vi "Get VI Property.vi"(8 "error in (no error)":errorcluster, 10 "VI Property":T1, 11 "VI Refnum in":refnum<vi>) -> (0 "error out":errorcluster, 1 "Supported?":bool, 2 "Value":string, 3 "VI Refnum out":refnum<vi>)   [LabVIEW 2019, in "Project Properties.lvlib"]
doc: "Returns the <b>VI Property</b> as a string value. <b>Supported?</b> returns True if the property is accessable.\n\nCreated by: Ryan Pacini"
uses:
  Project Properties.lvlib
  VI Property.ctl
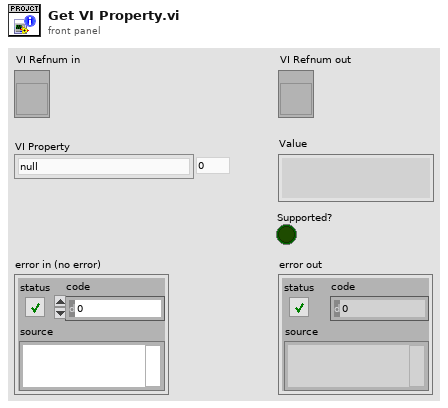
[diagram p1: front panel]
types:
  T1 = typedef "Project Properties.lvlib/VI Property.ctl" = enum8{"null", "Auto Logging:Log at Finish", "Auto Logging:Log File Path", "Auto Logging:Print at Finish", "Auto Preallocate Arrays and Strings", "Automatic Error Handling", "BD Master Wizard", "Block Diagram", "Block Diagram Window:Alignment Grid Size", "Block Diagram Window:Native Window", "Block Diagram Window:Open", "Block Diagram Window:Origin", "Block Diagram Window:State", "Block Diagram Window:Window Bounds", "Block Diagram Window:Window Interface", "Callers' Names", "Callers' Paths", "Compiled:Code Complexity", "Compiled:Last Compiled With", "Compiler:Generated Code Profiling Result", "Compiler:Generated Code Profiling Settings", "Connector Pane:Checksum Ignore Dynamic Dispatch v2", "Connector Pane:Checksum v3", "Connector Pane:DataType", "Connector Pane:Reference", "Connector Pane:Set", "Contains Compiled Code", "Context:Has Edits In Another Context", "Context:Has Edits In This Context", "Context:Is Reserved In Other Context", "Context:Is Reserved In This Context", "Control VI Type", "Did Recompile InThis Version", "Do Not Show Save Changes Dialog", "Edit Mode On Open", "Execution highlighting?", "Execution:Allow Debugging", "Execution:Close After Call", "Execution:Compiled With SSE", "Execution:Did Compiler Or User Approve Inlining", "Execution:Inline Enum", "Execution:Inline Is Allowed", "Execution:Inline SubVI", "Execution:Inline SubVI If Possible", "Execution:Is Reentrant", "Execution:Preferred Exec System", "Execution:Priority", "Execution:Reentrancy Type", "Execution:Retain Wire Values", "Execution:Run When Opened", "Execution:Show Front Panel On Call", "Execution:Show Front Panel On Load", "Execution:Shrink Large Buffer Threshold", "Execution:Shrink Large Buffers", "Execution:SSE Runtime Optimization", "Execution:State", "Execution:Suspend On Call", "Expand When Dropped As SubVI", "Front Panel", "Front Panel RefNum TD", "Front Panel Window:Alignment Grid Size", "Front Panel Window:Allow Runtime PopUp", "Front Panel Window:Behavior", "Front Panel Window:Closeable", "Front Panel Window:Custom Title", "Front Panel Window:Highlight Return Button", "Front Panel Window:Is Floating", "Front Panel Window:Is Frontmost", "Front Panel Window:Keep Window Proportions", "Front Panel Window:Minimizable", "Front Panel Window:Minimum Size", "Front Panel Window:Monitor", "Front Panel Window:Native Window", "Front Panel Window:Panel Bounds", "Front Panel Window:Resizable", "Front Panel Window:Run VI Transparently", "Front Panel Window:Show Menu Bar", "Front Panel Window:State", "Front Panel Window:Title", "Front Panel Window:Title Bar Visible", "Front Panel Window:Transparency", "Front Panel Window:Window Bounds", "Front Panel Window:Window Interface", "Has MathScript Nodes", "Help:Document Path", "Help:Document Tag", "Help:Document Web URL", "Help:Examples Exist", "Help:Use Web URL", "Hide Instance VI Caption On Drop", "History:Always Add Comments At Save", "History:Entire Text", "History:Prompt for Comments At Close", "History:Prompt for Comments At Save", "History:Record Application Comments", "History:Revision Number", "History:Use Defaults", "Inline Callees", "Is Clone VI", "Is Generic", "Is In Packed Library", "Is Instance", "Is Probe", "Is Running Interactively", "Is Skinned", "Is System VI", "Is VI Paused?", "Is XNode VI", "Item ID", "Ladder VI Needs Scripting", "Library", "Library:Private", "Library:Version", "Metrics:Advanced", "Metrics:Block Diagram Loaded", "Metrics:Code Size", "Metrics:Front Panel Loaded", "Metrics:Number of clones", "Metrics:Size of Block Diagram", "Metrics:Size of Front Panel", "Metrics:Total Data Size", "Modifications:Block Diagram Mods Bitset", "Modifications:Front Panel Mods Bitset", "Modifications:User Changes", "Modifications:VI Modifications Bitset", "Modifications:VI Signatures", "Modifications:VI User Code GUID", "No Clone If Instance VI", "Number of Non-Proxy Callers", "Overload Info", "Owning Application", "Printing:Block Diagram Scaling?", "Printing:Front Panel Scaling?", "Printing:Header Content:Date Printed?", "Printing:Header Content:Modify Date?", "Printing:Header Content:Page Number?", "Printing:Header Content:VI Icon?", "Printing:Header Content:VI Name?", "Printing:Header Content:VI Path?", "Printing:Margins", "Printing:Page Headers?", "Printing:Page Orientation", "Purgative", "Run-Time Menu Path", "Saved Version", "Statechart:Is Sub Panel Editable", "Statechart:Supress Parse", "Suppress Data Manager", "Suppress Instance VI Halo", "Suppress Transact Info", "Suppress Type Prop", "Tagged And Not Edited", "Terminal Bounds[]", "Tool Bar:Show Abort Button", "Tool Bar:Show Free Run Button", "Tool Bar:Show Run Button", "Tool Bar:Visible", "Tool Kit Attr", "VI Clone Name", "VI Compile Time", "VI Description", "VI Linker Errors", "VI Name", "VI Path", "VI Type"}
  T2 = typedef "LVPointTypeDef.ctl" = cluster{"Horizontal":i16, "Vertical":i16}
  T3 = enum32{"Invalid", "Standard", "Closed", "Hidden", "Minimized", "Maximized"}
  T4 = typedef "LVRectTypeDef.ctl" = cluster{"Left":i16, "Top":i16, "Right":i16, "Bottom":i16}
  T5 = typedef "LVLastCompiledWithTypeDef.ctl" = enum16{"Partial compiler optimizations", "Full compiler optimizations"}
  T6 = enum32{"not a control VI", "control", "typedef", "strict typedef"}
  T7 = enum32{"invalid execution system", "user interface", "standard", "instrument i/o", "data acquisition", "other 1", "other 2", "same as caller"}
  T8 = enum32{"invalid priority", "background priority", "normal priority", "above normal priority", "high priority", "time critical priority", "subroutine"}
  T9 = enum16{"Share clones between instances", "Preallocate clone for each instance"}
  T10 = enum32{"Bad", "Idle", "Run top level", "Running"}
  T11 = enum32{"Invalid", "Default", "Floating", "Floating/Auto-Hide", "Modal"}
  T12 = cluster{"Major":u16, "Minor":u16, "Fix":u16, "Build":u16}
  T13 = typedef "LVPrintingMarginsTypeDef.ctl" = cluster{"Top":sgl, "Left":sgl, "Bottom":sgl, "Right":sgl, "Measurement System":enum8{"Inches", "cm"}}
  T14 = enum32{"Portrait", "Landscape", "Rotated Portrait", "Rotated Landscape"}
  T15 = cluster{"Creator":string, "Toolkit":string, "Version":i32}
  T16 = enum32{"invalid VI type", "Standard VI", "Control VI", "Global VI", "Polymorphic VI", "Configuration VI", "SubSystem", "Facade VI", "Method VI", "Statechart Diagram VI"}
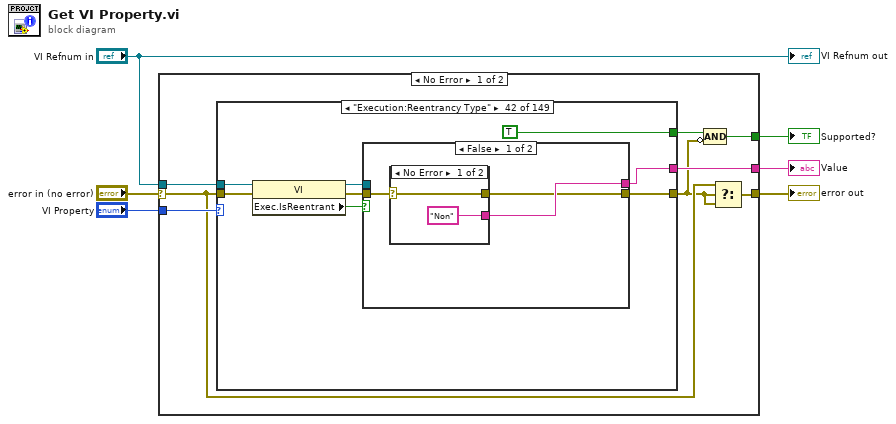
[diagram p0: block diagram]
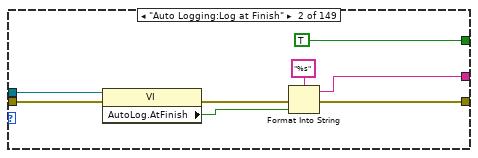
[diagram p3: hidden frame]
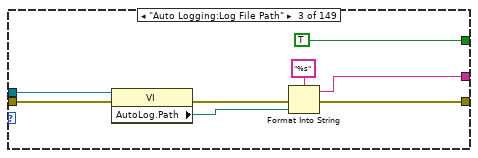
[diagram p4: hidden frame]
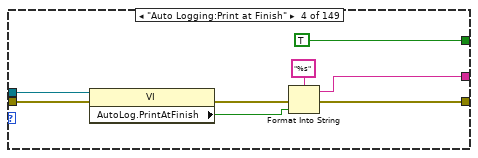
[diagram p5: hidden frame]
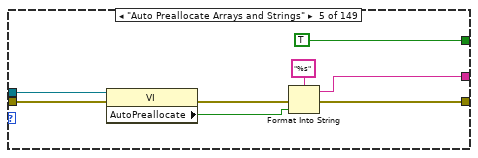
[diagram p6: hidden frame]
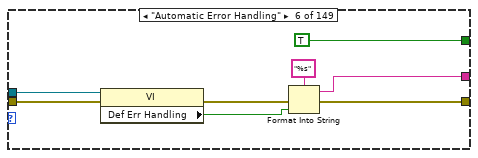
[diagram p7: hidden frame]
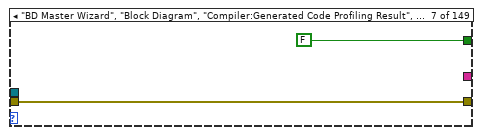
[diagram p8: hidden frame]
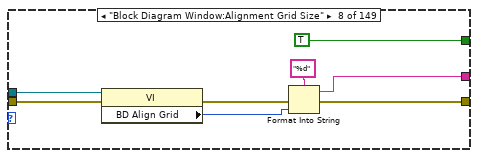
[diagram p9: hidden frame]
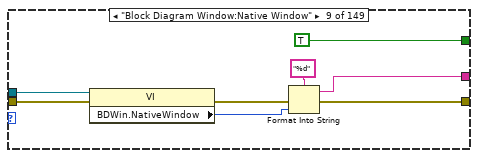
[diagram p10: hidden frame]
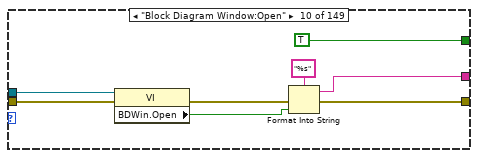
[diagram p11: hidden frame]
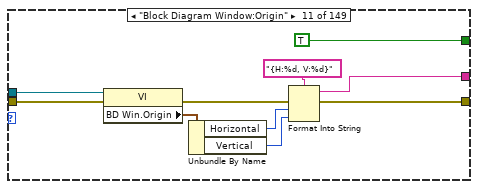
[diagram p12: hidden frame]
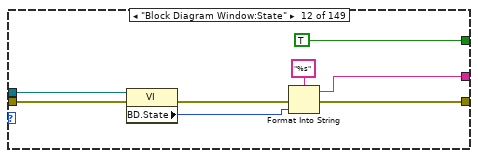
[diagram p13: hidden frame]
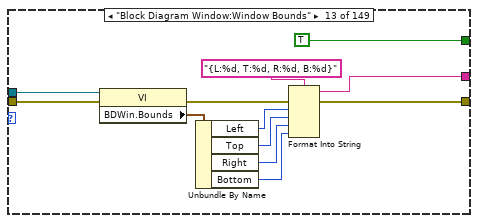
[diagram p14: hidden frame]
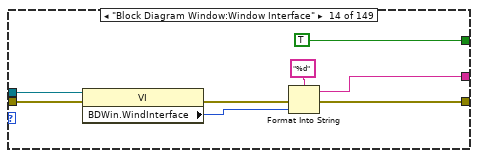
[diagram p15: hidden frame]
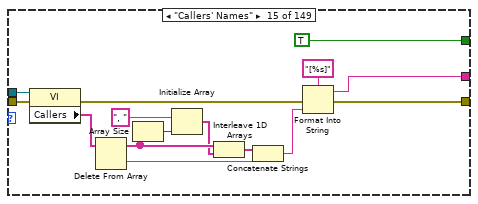
[diagram p16: hidden frame]
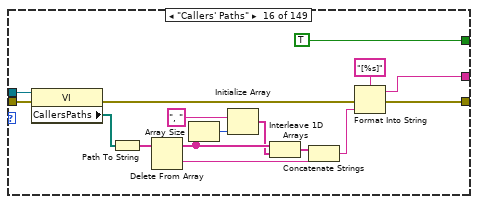
[diagram p17: hidden frame]
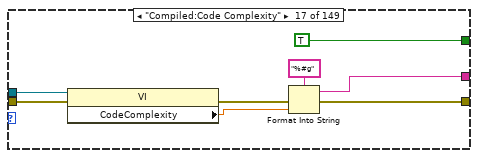
[diagram p18: hidden frame]
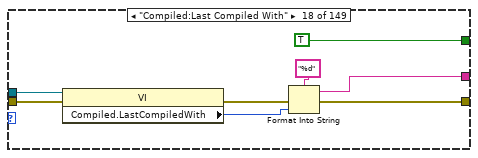
[diagram p19: hidden frame]
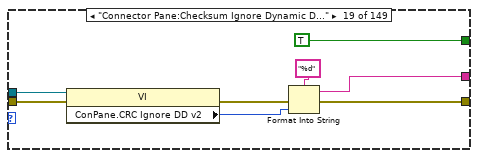
[diagram p20: hidden frame]
diagram:
  n1 = case shown="No Error" "error in (no error)" {
    selector: "error in (no error)" -> [w12 w1271]
    tunnel: "VI Property" -> [w14 _]
    tunnel: "VI Refnum in" -> [w13 _]
    tunnel: [w7 _] -> w3
    tunnel: [w11 w1271] -> w2
    tunnel: [w10 _] -> w1
    frame No Error {
      n2 = case shown="\"Execution:Reentrancy Type\"" w14 {
        tunnel: w12 -> [w15 w23 w31 w39 w47 w55 w56 w65 w73 w81 w91 w99 w111 w119 w134 w150 w158 w166 w174 w182 w190 w198 w206 w214 w222 w230 w238 w246 w254 w262 w270 w278 w286 w294 w302 w310 w318 w326 w334 w342 w350 w353 w382 w390 w398 w406 w414 w422 w430 w438 w446 w454 w462 w470 w478 w486 w494 w502 w510 w518 w526 w534 w544 w552 w560 w572 w580 w588 w596 w604 w612 w620 w628 w640 w648 w656 w664 w672 w680 w688 w696 w704 w712 w720 w728 w736 w744 w752 w760 w768 w776 w784 w792 w800 w808 w816 w824 w832 w840 w848 w856 w868 w876 w884 w892 w900 w908 w916 w924 w932 w940 w948 w956 w964 w972 w980 w988 w996 w1004 w1012 w1020 w1028 w1036 w1049 w1057 w1065 w1073 w1081 w1089 w1097 w1105 w1113 w1121 w1129 w1137 w1145 w1162 w1179 w1187 w1195 w1203 w1214 w1222 w1230 w1238 w1246 w1254 w1262 w1270]
        tunnel: w13 -> [_ w22 w30 w38 w46 w54 _ w64 w72 w80 w90 w98 w110 w118 w133 w149 w157 w165 w173 w181 w189 w197 w205 w213 w221 w229 w237 w245 w253 w261 w269 w277 w285 w293 w301 w309 w317 w325 w333 w341 w349 w358 w381 w389 w397 w405 w413 w421 w429 w437 w445 w453 w461 w469 w477 w485 w493 w501 w509 w517 w525 w533 w543 w551 w559 w571 w579 w587 w595 w603 w611 w619 w627 w639 w647 w655 w663 w671 w679 w687 w695 w703 w711 w719 w727 w735 w743 w751 w759 w767 w775 w783 w791 w799 w807 w815 w823 w831 w839 w847 w855 w867 w875 w883 w891 w899 w907 w915 w923 w931 w939 w947 w955 w963 w971 w979 w987 w995 w1003 w1011 w1019 w1027 w1035 w1048 w1056 w1064 w1072 w1080 w1088 w1096 w1104 w1112 w1120 w1128 w1136 w1144 w1161 w1178 w1186 w1194 w1202 w1213 w1221 w1229 w1237 w1245 w1253 w1261 w1269]
        tunnel: [w15 w19 w27 w35 w43 w51 w56 w61 w69 w77 w87 w95 w107 w115 w123 w138 w154 w162 w170 w178 w186 w194 w202 w210 w218 w226 w234 w242 w250 w258 w266 w274 w282 w290 w298 w306 w314 w322 w330 w338 w346 w356 w378 w386 w394 w402 w410 w418 w426 w434 w442 w450 w458 w466 w474 w482 w490 w498 w506 w514 w522 w530 w540 w548 w556 w568 w576 w584 w592 w600 w608 w616 w624 w636 w644 w652 w660 w668 w676 w684 w692 w700 w708 w716 w724 w732 w740 w748 w756 w764 w772 w780 w788 w796 w804 w812 w820 w828 w836 w844 w852 w864 w872 w880 w888 w896 w904 w912 w920 w928 w936 w944 w952 w960 w968 w976 w984 w992 w1000 w1008 w1016 w1024 w1032 w1045 w1053 w1061 w1069 w1077 w1085 w1093 w1101 w1109 w1117 w1125 w1133 w1141 w1150 w1175 w1183 w1191 w1199 w1210 w1218 w1226 w1234 w1242 w1250 w1258 w1266] -> w9
        tunnel: [_ TRUE TRUE TRUE TRUE TRUE FALSE TRUE TRUE TRUE TRUE TRUE TRUE TRUE TRUE TRUE TRUE TRUE TRUE TRUE TRUE TRUE TRUE TRUE TRUE TRUE TRUE TRUE TRUE TRUE TRUE TRUE TRUE TRUE TRUE TRUE TRUE TRUE TRUE TRUE TRUE TRUE TRUE TRUE TRUE TRUE TRUE TRUE TRUE TRUE TRUE TRUE TRUE TRUE TRUE TRUE TRUE TRUE TRUE TRUE TRUE TRUE TRUE TRUE TRUE TRUE TRUE TRUE TRUE TRUE TRUE TRUE TRUE TRUE TRUE TRUE TRUE TRUE TRUE TRUE TRUE TRUE TRUE TRUE TRUE TRUE TRUE TRUE TRUE TRUE TRUE TRUE TRUE TRUE TRUE TRUE TRUE TRUE TRUE TRUE TRUE TRUE TRUE TRUE TRUE TRUE TRUE TRUE TRUE TRUE TRUE TRUE TRUE TRUE TRUE TRUE TRUE TRUE TRUE TRUE TRUE TRUE TRUE TRUE TRUE TRUE TRUE TRUE TRUE TRUE TRUE TRUE TRUE TRUE TRUE TRUE TRUE TRUE TRUE TRUE TRUE TRUE TRUE TRUE TRUE TRUE TRUE TRUE TRUE] -> w8
        tunnel: [_ w16 w24 w32 w40 w48 _ w58 w66 w74 w85 w92 w105 w113 w121 w136 w152 w160 w168 w176 w184 w192 w200 w208 w216 w224 w232 w240 w248 w256 w264 w272 w280 w288 w296 w304 w312 w320 w328 w336 w344 w355 w376 w384 w392 w400 w408 w416 w424 w432 w440 w448 w456 w464 w472 w480 w488 w496 w504 w512 w520 w528 w538 w546 w554 w566 w574 w582 w590 w598 w606 w614 w622 w634 w642 w650 w658 w666 w674 w682 w690 w698 w706 w714 w722 w730 w738 w746 w754 w762 w770 w778 w786 w794 w802 w810 w818 w826 w834 w842 w850 w862 w870 w878 w886 w894 w902 w910 w918 w926 w934 w942 w950 w958 w966 w974 w982 w990 w998 w1006 w1014 w1022 w1030 w1043 w1051 w1059 w1067 w1075 w1083 w1091 w1099 w1107 w1115 w1123 w1131 w1139 w1148 w1173 w1181 w1189 w1197 w1208 w1216 w1224 w1232 w1240 w1248 w1256 w1264] -> w10
        frame "null" {
        }
        frame "Auto Logging:Log at Finish" {
          n3 = property class="VI"(reference=w22, error in=w23) -> (error out=w20:errorcluster, "AutoLog.AtFinish"=w18:bool)  [unwired: 1 out]
          n4 = Format Into String(format string="%s", error in=w20, w18) -> (resulting string=w16:string, error out=w19:errorcluster)  [unwired: 1 in]
        }
        frame "Auto Logging:Log File Path" {
          n5 = property class="VI"(reference=w30, error in=w31) -> (error out=w28:errorcluster, "AutoLog.Path"=w26:path)  [unwired: 1 out]
          n6 = Format Into String(format string="%s", error in=w28, w26) -> (resulting string=w24:string, error out=w27:errorcluster)  [unwired: 1 in]
        }
        frame "Auto Logging:Print at Finish" {
          n7 = property class="VI"(reference=w38, error in=w39) -> (error out=w36:errorcluster, "AutoLog.PrintAtFinish"=w34:bool)  [unwired: 1 out]
          n8 = Format Into String(format string="%s", error in=w36, w34) -> (resulting string=w32:string, error out=w35:errorcluster)  [unwired: 1 in]
        }
        frame "Auto Preallocate Arrays and Strings" {
          n9 = property class="VI"(reference=w46, error in=w47) -> (error out=w44:errorcluster, "AutoPreallocate"=w42:bool)  [unwired: 1 out]
          n10 = Format Into String(format string="%s", error in=w44, w42) -> (resulting string=w40:string, error out=w43:errorcluster)  [unwired: 1 in]
        }
        frame "Automatic Error Handling" {
          n11 = property class="VI"(reference=w54, error in=w55) -> (error out=w52:errorcluster, "Def Err Handling"=w50:bool)  [unwired: 1 out]
          n12 = Format Into String(format string="%s", error in=w52, w50) -> (resulting string=w48:string, error out=w51:errorcluster)  [unwired: 1 in]
        }
        frame "BD Master Wizard", "Block Diagram", "Compiler:Generated Code Profiling Result", "Compiler:Generated Code Profiling Settings", "Connector Pane:DataType".."Connector Pane:Set", "Front Panel", "Front Panel RefNum TD", "Inline Callees", "Library", "Library:Private", "Metrics:Advanced", "Modifications:VI Signatures", "Modifications:VI User Code GUID", "Overload Info", "Owning Application" {
        }
        frame "Block Diagram Window:Alignment Grid Size" {
          n13 = property class="VI"(reference=w64, error in=w65) -> (error out=w62:errorcluster, "BD Align Grid"=w60:i32)  [unwired: 1 out]
          n14 = Format Into String(format string="%d", error in=w62, w60) -> (resulting string=w58:string, error out=w61:errorcluster)  [unwired: 1 in]
        }
        frame "Block Diagram Window:Native Window" {
          n15 = property class="VI"(reference=w72, error in=w73) -> (error out=w70:errorcluster, "BDWin.NativeWindow"=w68:u64)  [unwired: 1 out]
          n16 = Format Into String(format string="%d", error in=w70, w68) -> (resulting string=w66:string, error out=w69:errorcluster)  [unwired: 1 in]
        }
        frame "Block Diagram Window:Open" {
          n17 = property class="VI"(reference=w80, error in=w81) -> (error out=w78:errorcluster, "BDWin.Open"=w76:bool)  [unwired: 1 out]
          n18 = Format Into String(format string="%s", error in=w78, w76) -> (resulting string=w74:string, error out=w77:errorcluster)  [unwired: 1 in]
        }
        frame "Block Diagram Window:Origin" {
          n19 = property class="VI"(reference=w90, error in=w91) -> (error out=w88:errorcluster, "BD Win.Origin"=w84:T2)  [unwired: 1 out]
          n20 = Unbundle By Name(w84) -> ("Horizontal"=w83:i16, "Vertical"=w82:i16)
          n21 = Format Into String(format string="{H:%d, V:%d}", error in=w88, w83, w82) -> (resulting string=w85:string, error out=w87:errorcluster)  [unwired: 1 in]
        }
        frame "Block Diagram Window:State" {
          n22 = property class="VI"(reference=w98, error in=w99) -> (error out=w96:errorcluster, "BD.State"=w94:T3)  [unwired: 1 out]
          n23 = Format Into String(format string="%s", error in=w96, w94) -> (resulting string=w92:string, error out=w95:errorcluster)  [unwired: 1 in]
        }
        frame "Block Diagram Window:Window Bounds" {
          n24 = property class="VI"(reference=w110, error in=w111) -> (error out=w108:errorcluster, "BDWin.Bounds"=w104:T4)  [unwired: 1 out]
          n25 = Unbundle By Name(w104) -> ("Left"=w103:i16, "Top"=w102:i16, "Right"=w101:i16, "Bottom"=w100:i16)
          n26 = Format Into String(format string="{L:%d, T:%d, R:%d, B:%d}", error in=w108, w103, w102, w101, w100) -> (resulting string=w105:string, error out=w107:errorcluster)  [unwired: 1 in]
        }
        frame "Block Diagram Window:Window Interface" {
          n27 = property class="VI"(reference=w118, error in=w119) -> (error out=w116:errorcluster, "BDWin.WindInterface"=w112:u64)  [unwired: 1 out]
          n28 = Format Into String(format string="%d", error in=w116, w112) -> (resulting string=w113:string, error out=w115:errorcluster)  [unwired: 1 in]
        }
        frame "Callers' Names" {
          n29 = property class="VI"(reference=w133, error in=w134) -> (error out=w124:errorcluster, "Callers"=w129:string[])  [unwired: 1 out]
          n30 = Delete From Array(array=w129) -> (deleted portion=w125:string, array with subset deleted=w128:string[])  [unwired: 2 in]
          n31 = Array Size(array=w128) -> (size(s)=w131:i32)
          n32 = Initialize Array(", ", w131) -> (w127:string[])
          n33 = Interleave 1D Arrays(w128, w127) -> (w126:string[])
          n34 = Concatenate Strings(w126, w125) -> (w122:string)
          n35 = Format Into String(format string="[%s]", error in=w124, w122) -> (resulting string=w121:string, error out=w123:errorcluster)  [unwired: 1 in]
        }
        frame "Callers' Paths" {
          n36 = property class="VI"(reference=w149, error in=w150) -> (error out=w140:errorcluster, "CallersPaths"=w145:path[])  [unwired: 1 out]
          n37 = Path To String(path=w145) -> (string=w139:string[])
          n38 = Delete From Array(array=w139) -> (deleted portion=w141:string, array with subset deleted=w144:string[])  [unwired: 2 in]
          n39 = Array Size(array=w144) -> (size(s)=w147:i32)
          n40 = Initialize Array(", ", w147) -> (w143:string[])
          n41 = Interleave 1D Arrays(w144, w143) -> (w142:string[])
          n42 = Concatenate Strings(w142, w141) -> (w137:string)
          n43 = Format Into String(format string="[%s]", error in=w140, w137) -> (resulting string=w136:string, error out=w138:errorcluster)  [unwired: 1 in]
        }
        frame "Compiled:Code Complexity" {
          n44 = property class="VI"(reference=w157, error in=w158) -> (error out=w155:errorcluster, "CodeComplexity"=w151:sgl)  [unwired: 1 out]
          n45 = Format Into String(format string="%#g", error in=w155, w151) -> (resulting string=w152:string, error out=w154:errorcluster)  [unwired: 1 in]
        }
        frame "Compiled:Last Compiled With" {
          n46 = property class="VI"(reference=w165, error in=w166) -> (error out=w163:errorcluster, "Compiled.LastCompiledWith"=w159:T5)  [unwired: 1 out]
          n47 = Format Into String(format string="%d", error in=w163, w159) -> (resulting string=w160:string, error out=w162:errorcluster)  [unwired: 1 in]
        }
        frame "Connector Pane:Checksum Ignore Dynamic Dispatch v2" {
          n48 = property class="VI"(reference=w173, error in=w174) -> (error out=w171:errorcluster, "ConPane.CRC Ignore DD v2"=w167:i32)  [unwired: 1 out]
          n49 = Format Into String(format string="%d", error in=w171, w167) -> (resulting string=w168:string, error out=w170:errorcluster)  [unwired: 1 in]
        }
        frame "Connector Pane:Checksum v3" {
          n50 = property class="VI"(reference=w181, error in=w182) -> (error out=w179:errorcluster, "ConPane.CRC v3"=w175:i32)  [unwired: 1 out]
          n51 = Format Into String(format string="%d", error in=w179, w175) -> (resulting string=w176:string, error out=w178:errorcluster)  [unwired: 1 in]
        }
        frame "Contains Compiled Code" {
          n52 = property class="VI"(reference=w189, error in=w190) -> (error out=w187:errorcluster, "ContainstCompiledCode"=w183:bool)  [unwired: 1 out]
          n53 = Format Into String(format string="%s", error in=w187, w183) -> (resulting string=w184:string, error out=w186:errorcluster)  [unwired: 1 in]
        }
        frame "Context:Has Edits In Another Context" {
          n54 = property class="VI"(reference=w197, error in=w198) -> (error out=w195:errorcluster, "HasEditsInAnotherContext"=w191:bool)  [unwired: 1 out]
          n55 = Format Into String(format string="%s", error in=w195, w191) -> (resulting string=w192:string, error out=w194:errorcluster)  [unwired: 1 in]
        }
        frame "Context:Has Edits In This Context" {
          n56 = property class="VI"(reference=w205, error in=w206) -> (error out=w203:errorcluster, "HasEditsInThisContext"=w199:bool)  [unwired: 1 out]
          n57 = Format Into String(format string="%s", error in=w203, w199) -> (resulting string=w200:string, error out=w202:errorcluster)  [unwired: 1 in]
        }
        frame "Context:Is Reserved In Other Context" {
          n58 = property class="VI"(reference=w213, error in=w214) -> (error out=w211:errorcluster, "IsReservedInOtherContext"=w207:bool)  [unwired: 1 out]
          n59 = Format Into String(format string="%s", error in=w211, w207) -> (resulting string=w208:string, error out=w210:errorcluster)  [unwired: 1 in]
        }
        frame "Context:Is Reserved In This Context" {
          n60 = property class="VI"(reference=w221, error in=w222) -> (error out=w219:errorcluster, "IsReservedInThisContext"=w215:bool)  [unwired: 1 out]
          n61 = Format Into String(format string="%s", error in=w219, w215) -> (resulting string=w216:string, error out=w218:errorcluster)  [unwired: 1 in]
        }
        frame "Control VI Type" {
          n62 = property class="VI"(reference=w229, error in=w230) -> (error out=w227:errorcluster, "CtrlVIType"=w223:T6)  [unwired: 1 out]
          n63 = Format Into String(format string="%s", error in=w227, w223) -> (resulting string=w224:string, error out=w226:errorcluster)  [unwired: 1 in]
        }
        frame "Did Recompile InThis Version" {
          n64 = property class="VI"(reference=w237, error in=w238) -> (error out=w235:errorcluster, "DidRecompileInThisVersion"=w231:bool)  [unwired: 1 out]
          n65 = Format Into String(format string="%s", error in=w235, w231) -> (resulting string=w232:string, error out=w234:errorcluster)  [unwired: 1 in]
        }
        frame "Do Not Show Save Changes Dialog" {
          n66 = property class="VI"(reference=w245, error in=w246) -> (error out=w243:errorcluster, "DoNotShowSaveChangesDialog"=w239:bool)  [unwired: 1 out]
          n67 = Format Into String(format string="%s", error in=w243, w239) -> (resulting string=w240:string, error out=w242:errorcluster)  [unwired: 1 in]
        }
        frame "Edit Mode On Open" {
          n68 = property class="VI"(reference=w253, error in=w254) -> (error out=w251:errorcluster, "Edit Mode"=w247:bool)  [unwired: 1 out]
          n69 = Format Into String(format string="%s", error in=w251, w247) -> (resulting string=w248:string, error out=w250:errorcluster)  [unwired: 1 in]
        }
        frame "Execution highlighting?" {
          n70 = property class="VI"(reference=w261, error in=w262) -> (error out=w259:errorcluster, "Highlight?"=w255:bool)  [unwired: 1 out]
          n71 = Format Into String(format string="%s", error in=w259, w255) -> (resulting string=w256:string, error out=w258:errorcluster)  [unwired: 1 in]
        }
        frame "Execution:Allow Debugging" {
          n72 = property class="VI"(reference=w269, error in=w270) -> (error out=w267:errorcluster, "Exec.AllowDebug"=w263:bool)  [unwired: 1 out]
          n73 = Format Into String(format string="%s", error in=w267, w263) -> (resulting string=w264:string, error out=w266:errorcluster)  [unwired: 1 in]
        }
        frame "Execution:Close After Call" {
          n74 = property class="VI"(reference=w277, error in=w278) -> (error out=w275:errorcluster, "Exec.CloseFPAfterCall"=w271:bool)  [unwired: 1 out]
          n75 = Format Into String(format string="%s", error in=w275, w271) -> (resulting string=w272:string, error out=w274:errorcluster)  [unwired: 1 in]
        }
        frame "Execution:Compiled With SSE" {
          n76 = property class="VI"(reference=w285, error in=w286) -> (error out=w283:errorcluster, "ExecCompiledWithSSE"=w279:bool)  [unwired: 1 out]
          n77 = Format Into String(format string="%s", error in=w283, w279) -> (resulting string=w280:string, error out=w282:errorcluster)  [unwired: 1 in]
        }
        frame "Execution:Did Compiler Or User Approve Inlining" {
          n78 = property class="VI"(reference=w293, error in=w294) -> (error out=w291:errorcluster, "Exec.DidCompilerOrUserApproveInlining"=w287:bool)  [unwired: 1 out]
          n79 = Format Into String(format string="%s", error in=w291, w287) -> (resulting string=w288:string, error out=w290:errorcluster)  [unwired: 1 in]
        }
        frame "Execution:Inline Enum" {
          n80 = property class="VI"(reference=w301, error in=w302) -> (error out=w299:errorcluster, "Exec.InlineSubVIEnum"=w295:u32)  [unwired: 1 out]
          n81 = Format Into String(format string="%d", error in=w299, w295) -> (resulting string=w296:string, error out=w298:errorcluster)  [unwired: 1 in]
        }
        frame "Execution:Inline Is Allowed" {
          n82 = property class="VI"(reference=w309, error in=w310) -> (error out=w307:errorcluster, "ExecIsInlineable"=w303:bool)  [unwired: 1 out]
          n83 = Format Into String(format string="%s", error in=w307, w303) -> (resulting string=w304:string, error out=w306:errorcluster)  [unwired: 1 in]
        }
        frame "Execution:Inline SubVI" {
          n84 = property class="VI"(reference=w317, error in=w318) -> (error out=w315:errorcluster, "ExecInlining"=w311:bool)  [unwired: 1 out]
          n85 = Format Into String(format string="%s", error in=w315, w311) -> (resulting string=w312:string, error out=w314:errorcluster)  [unwired: 1 in]
        }
        frame "Execution:Inline SubVI If Possible" {
          n86 = property class="VI"(reference=w325, error in=w326) -> (error out=w323:errorcluster, "ExecInlineIfPossible"=w319:bool)  [unwired: 1 out]
          n87 = Format Into String(format string="%s", error in=w323, w319) -> (resulting string=w320:string, error out=w322:errorcluster)  [unwired: 1 in]
        }
        frame "Execution:Is Reentrant" {
          n88 = property class="VI"(reference=w333, error in=w334) -> (error out=w331:errorcluster, "Exec.IsReentrant"=w327:bool)  [unwired: 1 out]
          n89 = Format Into String(format string="%s", error in=w331, w327) -> (resulting string=w328:string, error out=w330:errorcluster)  [unwired: 1 in]
        }
        frame "Execution:Preferred Exec System" {
          n90 = property class="VI"(reference=w341, error in=w342) -> (error out=w339:errorcluster, "Exec.PrefSys"=w335:T7)  [unwired: 1 out]
          n91 = Format Into String(format string="%s", error in=w339, w335) -> (resulting string=w336:string, error out=w338:errorcluster)  [unwired: 1 in]
        }
        frame "Execution:Priority" {
          n92 = property class="VI"(reference=w349, error in=w350) -> (error out=w347:errorcluster, "Exec.Priority"=w343:T8)  [unwired: 1 out]
          n93 = Format Into String(format string="%s", error in=w347, w343) -> (resulting string=w344:string, error out=w346:errorcluster)  [unwired: 1 in]
        }
        frame "Execution:Reentrancy Type" {
          n94 = property class="VI"(reference=w358, error in=w353) -> (reference out=w354:refnum<vi>, error out=w352:errorcluster, "Exec.IsReentrant"=w351:bool)
          n95 = case shown="False" w351 {
            tunnel: w352 -> [w359 w372]
            tunnel: w354 -> [_ w371]
            tunnel: [w360 w369] -> w356
            tunnel: [w361 w367] -> w355
            frame False {
              n96 = case shown="No Error" w359 {
                selector: w359 -> [w362 w364]
                tunnel: ["Non" _] -> w361
                tunnel: [w362 w364] -> w360
                frame No Error {
                }
                frame Error {
                }
              }
            }
            frame True {
              n97 = property class="VI"(reference=w371, error in=w372) -> (error out=w370:errorcluster, "Exec.ReentrancyType"=w366:T9)  [unwired: 1 out]
              n98 = case shown="\"Share clones between instances\"" w366 {
                tunnel: ["Share" ("format string") "Preallocate" ("format string")] -> w365
                frame "Share clones between instances" {
                }
                frame "Preallocate clone for each instance" {
                }
              }
              n99 = Format Into String(format string="%s", error in=w370, w365) -> (resulting string=w367:string, error out=w369:errorcluster)  [unwired: 1 in]
            }
          }
        }
        frame "Execution:Retain Wire Values" {
          n100 = property class="VI"(reference=w381, error in=w382) -> (error out=w379:errorcluster, "Exec.PostExecutionProbes"=w375:bool)  [unwired: 1 out]
          n101 = Format Into String(format string="%s", error in=w379, w375) -> (resulting string=w376:string, error out=w378:errorcluster)  [unwired: 1 in]
        }
        frame "Execution:Run When Opened" {
          n102 = property class="VI"(reference=w389, error in=w390) -> (error out=w387:errorcluster, "Exec.RunOnOpen"=w383:bool)  [unwired: 1 out]
          n103 = Format Into String(format string="%s", error in=w387, w383) -> (resulting string=w384:string, error out=w386:errorcluster)  [unwired: 1 in]
        }
        frame "Execution:Show Front Panel On Call" {
          n104 = property class="VI"(reference=w397, error in=w398) -> (error out=w395:errorcluster, "Exec.ShowFPOnCall"=w391:bool)  [unwired: 1 out]
          n105 = Format Into String(format string="%s", error in=w395, w391) -> (resulting string=w392:string, error out=w394:errorcluster)  [unwired: 1 in]
        }
        frame "Execution:Show Front Panel On Load" {
          n106 = property class="VI"(reference=w405, error in=w406) -> (error out=w403:errorcluster, "Exec.ShowFPOnLoad"=w399:bool)  [unwired: 1 out]
          n107 = Format Into String(format string="%s", error in=w403, w399) -> (resulting string=w400:string, error out=w402:errorcluster)  [unwired: 1 in]
        }
        frame "Execution:Shrink Large Buffer Threshold" {
          n108 = property class="VI"(reference=w413, error in=w414) -> (error out=w411:errorcluster, "Exec.ShrinkLargeBuffersThreshold"=w407:i32)  [unwired: 1 out]
          n109 = Format Into String(format string="%d", error in=w411, w407) -> (resulting string=w408:string, error out=w410:errorcluster)  [unwired: 1 in]
        }
        frame "Execution:Shrink Large Buffers" {
          n110 = property class="VI"(reference=w421, error in=w422) -> (error out=w419:errorcluster, "Exec.ShrinkLargeBuffers"=w415:bool)  [unwired: 1 out]
          n111 = Format Into String(format string="%s", error in=w419, w415) -> (resulting string=w416:string, error out=w418:errorcluster)  [unwired: 1 in]
        }
        frame "Execution:SSE Runtime Optimization" {
          n112 = property class="VI"(reference=w429, error in=w430) -> (error out=w427:errorcluster, "ExecSSERuntimeOptimization"=w423:bool)  [unwired: 1 out]
          n113 = Format Into String(format string="%s", error in=w427, w423) -> (resulting string=w424:string, error out=w426:errorcluster)  [unwired: 1 in]
        }
        frame "Execution:State" {
          n114 = property class="VI"(reference=w437, error in=w438) -> (error out=w435:errorcluster, "Exec.State"=w431:T10)  [unwired: 1 out]
          n115 = Format Into String(format string="%s", error in=w435, w431) -> (resulting string=w432:string, error out=w434:errorcluster)  [unwired: 1 in]
        }
        frame "Execution:Suspend On Call" {
          n116 = property class="VI"(reference=w445, error in=w446) -> (error out=w443:errorcluster, "Exec.SuspOnCall"=w439:bool)  [unwired: 1 out]
          n117 = Format Into String(format string="%s", error in=w443, w439) -> (resulting string=w440:string, error out=w442:errorcluster)  [unwired: 1 in]
        }
        frame "Expand When Dropped As SubVI" {
          n118 = property class="VI"(reference=w453, error in=w454) -> (error out=w451:errorcluster, "GrowByDefault"=w447:bool)  [unwired: 1 out]
          n119 = Format Into String(format string="%s", error in=w451, w447) -> (resulting string=w448:string, error out=w450:errorcluster)  [unwired: 1 in]
        }
        frame "Front Panel Window:Alignment Grid Size" {
          n120 = property class="VI"(reference=w461, error in=w462) -> (error out=w459:errorcluster, "FP Align Grid"=w455:i32)  [unwired: 1 out]
          n121 = Format Into String(format string="%d", error in=w459, w455) -> (resulting string=w456:string, error out=w458:errorcluster)  [unwired: 1 in]
        }
        frame "Front Panel Window:Allow Runtime PopUp" {
          n122 = property class="VI"(reference=w469, error in=w470) -> (error out=w467:errorcluster, "Front Panel.AllowRTPopup"=w463:bool)  [unwired: 1 out]
          n123 = Format Into String(format string="%d", error in=w467, w463) -> (resulting string=w464:string, error out=w466:errorcluster)  [unwired: 1 in]
        }
        frame "Front Panel Window:Behavior" {
          n124 = property class="VI"(reference=w477, error in=w478) -> (error out=w475:errorcluster, "FP.Behavior"=w471:T11)  [unwired: 1 out]
          n125 = Format Into String(format string="%d", error in=w475, w471) -> (resulting string=w472:string, error out=w474:errorcluster)  [unwired: 1 in]
        }
        frame "Front Panel Window:Closeable" {
          n126 = property class="VI"(reference=w485, error in=w486) -> (error out=w483:errorcluster, "Front Panel.Closeable"=w479:bool)  [unwired: 1 out]
          n127 = Format Into String(format string="%s", error in=w483, w479) -> (resulting string=w480:string, error out=w482:errorcluster)  [unwired: 1 in]
        }
        frame "Front Panel Window:Custom Title" {
          n128 = property class="VI"(reference=w493, error in=w494) -> (error out=w491:errorcluster, "Front Panel.CustomTitle"=w487:bool)  [unwired: 1 out]
          n129 = Format Into String(format string="%s", error in=w491, w487) -> (resulting string=w488:string, error out=w490:errorcluster)  [unwired: 1 in]
        }
        frame "Front Panel Window:Highlight Return Button" {
          n130 = property class="VI"(reference=w501, error in=w502) -> (error out=w499:errorcluster, "Front Panel.HiliteReturnBut"=w495:bool)  [unwired: 1 out]
          n131 = Format Into String(format string="%s", error in=w499, w495) -> (resulting string=w496:string, error out=w498:errorcluster)  [unwired: 1 in]
        }
        frame "Front Panel Window:Is Floating" {
          n132 = property class="VI"(reference=w509, error in=w510) -> (error out=w507:errorcluster, "FP.IsFloater"=w503:bool)  [unwired: 1 out]
          n133 = Format Into String(format string="%s", error in=w507, w503) -> (resulting string=w504:string, error out=w506:errorcluster)  [unwired: 1 in]
        }
        frame "Front Panel Window:Is Frontmost" {
          n134 = property class="VI"(reference=w517, error in=w518) -> (error out=w515:errorcluster, "Front Panel.IsFrontmost"=w511:bool)  [unwired: 1 out]
          n135 = Format Into String(format string="%s", error in=w515, w511) -> (resulting string=w512:string, error out=w514:errorcluster)  [unwired: 1 in]
        }
        frame "Front Panel Window:Keep Window Proportions" {
          n136 = property class="VI"(reference=w525, error in=w526) -> (error out=w523:errorcluster, "Front Panel.KeepWinProps"=w519:bool)  [unwired: 1 out]
          n137 = Format Into String(format string="%s", error in=w523, w519) -> (resulting string=w520:string, error out=w522:errorcluster)  [unwired: 1 in]
        }
        frame "Front Panel Window:Minimizable" {
          n138 = property class="VI"(reference=w533, error in=w534) -> (error out=w531:errorcluster, "Front Panel.Minimizeable"=w527:bool)  [unwired: 1 out]
          n139 = Format Into String(format string="%s", error in=w531, w527) -> (resulting string=w528:string, error out=w530:errorcluster)  [unwired: 1 in]
        }
        frame "Front Panel Window:Minimum Size" {
          n140 = property class="VI"(reference=w543, error in=w544) -> (error out=w541:errorcluster, "Minimum Panel Size"=w537:T2)  [unwired: 1 out]
          n141 = Unbundle By Name(w537) -> ("Horizontal"=w536:i16, "Vertical"=w535:i16)
          n142 = Format Into String(format string="{H:%d, V:%d}", error in=w541, w536, w535) -> (resulting string=w538:string, error out=w540:errorcluster)  [unwired: 1 in]
        }
        frame "Front Panel Window:Monitor" {
          n143 = property class="VI"(reference=w551, error in=w552) -> (error out=w549:errorcluster, "FP.Monitor"=w545:u16)  [unwired: 1 out]
          n144 = Format Into String(format string="%d", error in=w549, w545) -> (resulting string=w546:string, error out=w548:errorcluster)  [unwired: 1 in]
        }
        frame "Front Panel Window:Native Window" {
          n145 = property class="VI"(reference=w559, error in=w560) -> (error out=w557:errorcluster, "FP.NativeWindow"=w553:u64)  [unwired: 1 out]
          n146 = Format Into String(format string="%d", error in=w557, w553) -> (resulting string=w554:string, error out=w556:errorcluster)  [unwired: 1 in]
        }
        frame "Front Panel Window:Panel Bounds" {
          n147 = property class="VI"(reference=w571, error in=w572) -> (error out=w569:errorcluster, "Front Panel.PanelBounds"=w565:T4)  [unwired: 1 out]
          n148 = Unbundle By Name(w565) -> ("Left"=w564:i16, "Top"=w563:i16, "Right"=w562:i16, "Bottom"=w561:i16)
          n149 = Format Into String(format string="{L:%d, T:%d, R:%d, B:%d}", error in=w569, w564, w563, w562, w561) -> (resulting string=w566:string, error out=w568:errorcluster)  [unwired: 1 in]
        }
        frame "Front Panel Window:Resizable" {
          n150 = property class="VI"(reference=w579, error in=w580) -> (error out=w577:errorcluster, "Front Panel.Resizeable"=w573:bool)  [unwired: 1 out]
          n151 = Format Into String(format string="%s", error in=w577, w573) -> (resulting string=w574:string, error out=w576:errorcluster)  [unwired: 1 in]
        }
        frame "Front Panel Window:Run VI Transparently" {
          n152 = property class="VI"(reference=w587, error in=w588) -> (error out=w585:errorcluster, "FP:RunTransparently"=w581:bool)  [unwired: 1 out]
          n153 = Format Into String(format string="%s", error in=w585, w581) -> (resulting string=w582:string, error out=w584:errorcluster)  [unwired: 1 in]
        }
        frame "Front Panel Window:Show Menu Bar" {
          n154 = property class="VI"(reference=w595, error in=w596) -> (error out=w593:errorcluster, "Front Panel.ShowMenuBar"=w589:bool)  [unwired: 1 out]
          n155 = Format Into String(format string="%s", error in=w593, w589) -> (resulting string=w590:string, error out=w592:errorcluster)  [unwired: 1 in]
        }
        frame "Front Panel Window:State" {
          n156 = property class="VI"(reference=w603, error in=w604) -> (error out=w601:errorcluster, "FP.State"=w597:T3)  [unwired: 1 out]
          n157 = Format Into String(format string="%s", error in=w601, w597) -> (resulting string=w598:string, error out=w600:errorcluster)  [unwired: 1 in]
        }
        frame "Front Panel Window:Title" {
          n158 = property class="VI"(reference=w611, error in=w612) -> (error out=w609:errorcluster, "Front Panel.Title"=w605:string)  [unwired: 1 out]
          n159 = Format Into String(format string="%s", error in=w609, w605) -> (resulting string=w606:string, error out=w608:errorcluster)  [unwired: 1 in]
        }
        frame "Front Panel Window:Title Bar Visible" {
          n160 = property class="VI"(reference=w619, error in=w620) -> (error out=w617:errorcluster, "Front Panel.TitleBarVis"=w613:bool)  [unwired: 1 out]
          n161 = Format Into String(format string="%s", error in=w617, w613) -> (resulting string=w614:string, error out=w616:errorcluster)  [unwired: 1 in]
        }
        frame "Front Panel Window:Transparency" {
          n162 = property class="VI"(reference=w627, error in=w628) -> (error out=w625:errorcluster, "FP:Transparency"=w621:u8)  [unwired: 1 out]
          n163 = Format Into String(format string="%d", error in=w625, w621) -> (resulting string=w622:string, error out=w624:errorcluster)  [unwired: 1 in]
        }
        frame "Front Panel Window:Window Bounds" {
          n164 = property class="VI"(reference=w639, error in=w640) -> (error out=w637:errorcluster, "Front Panel.WinBounds"=w633:T4)  [unwired: 1 out]
          n165 = Unbundle By Name(w633) -> ("Left"=w632:i16, "Top"=w631:i16, "Right"=w630:i16, "Bottom"=w629:i16)
          n166 = Format Into String(format string="{L:%d, T:%d, R:%d, B:%d}", error in=w637, w632, w631, w630, w629) -> (resulting string=w634:string, error out=w636:errorcluster)  [unwired: 1 in]
        }
        frame "Front Panel Window:Window Interface" {
          n167 = property class="VI"(reference=w647, error in=w648) -> (error out=w645:errorcluster, "FP.WindInterface"=w641:u64)  [unwired: 1 out]
          n168 = Format Into String(format string="%d", error in=w645, w641) -> (resulting string=w642:string, error out=w644:errorcluster)  [unwired: 1 in]
        }
        frame "Has MathScript Nodes" {
          n169 = property class="VI"(reference=w655, error in=w656) -> (error out=w653:errorcluster, "HasMSN"=w649:bool)  [unwired: 1 out]
          n170 = Format Into String(format string="%s", error in=w653, w649) -> (resulting string=w650:string, error out=w652:errorcluster)  [unwired: 1 in]
        }
        frame "Help:Document Path" {
          n171 = property class="VI"(reference=w663, error in=w664) -> (error out=w661:errorcluster, "Help.Path"=w657:path)  [unwired: 1 out]
          n172 = Format Into String(format string="%s", error in=w661, w657) -> (resulting string=w658:string, error out=w660:errorcluster)  [unwired: 1 in]
        }
        frame "Help:Document Tag" {
          n173 = property class="VI"(reference=w671, error in=w672) -> (error out=w669:errorcluster, "Help.Tag"=w665:string)  [unwired: 1 out]
          n174 = Format Into String(format string="%s", error in=w669, w665) -> (resulting string=w666:string, error out=w668:errorcluster)  [unwired: 1 in]
        }
        frame "Help:Document Web URL" {
          n175 = property class="VI"(reference=w679, error in=w680) -> (error out=w677:errorcluster, "Help.URL"=w673:string)  [unwired: 1 out]
          n176 = Format Into String(format string="%s", error in=w677, w673) -> (resulting string=w674:string, error out=w676:errorcluster)  [unwired: 1 in]
        }
        frame "Help:Examples Exist" {
          n177 = property class="VI"(reference=w687, error in=w688) -> (error out=w685:errorcluster, "Help.Examples"=w681:bool)  [unwired: 1 out]
          n178 = Format Into String(format string="%s", error in=w685, w681) -> (resulting string=w682:string, error out=w684:errorcluster)  [unwired: 1 in]
        }
        frame "Help:Use Web URL" {
          n179 = property class="VI"(reference=w695, error in=w696) -> (error out=w693:errorcluster, "Help.UseOnline"=w689:bool)  [unwired: 1 out]
          n180 = Format Into String(format string="%s", error in=w693, w689) -> (resulting string=w690:string, error out=w692:errorcluster)  [unwired: 1 in]
        }
        frame "Hide Instance VI Caption On Drop" {
          n181 = property class="VI"(reference=w703, error in=w704) -> (error out=w701:errorcluster, "HideInstanceVICaptionOnDrop"=w697:bool)  [unwired: 1 out]
          n182 = Format Into String(format string="%s", error in=w701, w697) -> (resulting string=w698:string, error out=w700:errorcluster)  [unwired: 1 in]
        }
        frame "History:Always Add Comments At Save" {
          n183 = property class="VI"(reference=w711, error in=w712) -> (error out=w709:errorcluster, "Hist.AddAtSave"=w705:bool)  [unwired: 1 out]
          n184 = Format Into String(format string="%s", error in=w709, w705) -> (resulting string=w706:string, error out=w708:errorcluster)  [unwired: 1 in]
        }
        frame "History:Entire Text" {
          n185 = property class="VI"(reference=w719, error in=w720) -> (error out=w717:errorcluster, "Hist.Text"=w713:string)  [unwired: 1 out]
          n186 = Format Into String(format string="%s", error in=w717, w713) -> (resulting string=w714:string, error out=w716:errorcluster)  [unwired: 1 in]
        }
        frame "History:Prompt for Comments At Close" {
          n187 = property class="VI"(reference=w727, error in=w728) -> (error out=w725:errorcluster, "Hist.PromptAtClose"=w721:bool)  [unwired: 1 out]
          n188 = Format Into String(format string="%s", error in=w725, w721) -> (resulting string=w722:string, error out=w724:errorcluster)  [unwired: 1 in]
        }
        frame "History:Prompt for Comments At Save" {
          n189 = property class="VI"(reference=w735, error in=w736) -> (error out=w733:errorcluster, "Hist.PrompAtSave"=w729:bool)  [unwired: 1 out]
          n190 = Format Into String(format string="%s", error in=w733, w729) -> (resulting string=w730:string, error out=w732:errorcluster)  [unwired: 1 in]
        }
        frame "History:Record Application Comments" {
          n191 = property class="VI"(reference=w743, error in=w744) -> (error out=w741:errorcluster, "Hist.RecAppComments"=w737:bool)  [unwired: 1 out]
          n192 = Format Into String(format string="%s", error in=w741, w737) -> (resulting string=w738:string, error out=w740:errorcluster)  [unwired: 1 in]
        }
        frame "History:Revision Number" {
          n193 = property class="VI"(reference=w751, error in=w752) -> (error out=w749:errorcluster, "Hist.Revision"=w745:u32)  [unwired: 1 out]
          n194 = Format Into String(format string="%d", error in=w749, w745) -> (resulting string=w746:string, error out=w748:errorcluster)  [unwired: 1 in]
        }
        frame "History:Use Defaults" {
          n195 = property class="VI"(reference=w759, error in=w760) -> (error out=w757:errorcluster, "Hist.UseDflt"=w753:bool)  [unwired: 1 out]
          n196 = Format Into String(format string="%s", error in=w757, w753) -> (resulting string=w754:string, error out=w756:errorcluster)  [unwired: 1 in]
        }
        frame "Is Clone VI" {
          n197 = property class="VI"(reference=w767, error in=w768) -> (error out=w765:errorcluster, "IsCloneVI"=w761:bool)  [unwired: 1 out]
          n198 = Format Into String(format string="%s", error in=w765, w761) -> (resulting string=w762:string, error out=w764:errorcluster)  [unwired: 1 in]
        }
        frame "Is Generic" {
          n199 = property class="VI"(reference=w775, error in=w776) -> (error out=w773:errorcluster, "IsGeneric"=w769:bool)  [unwired: 1 out]
          n200 = Format Into String(format string="%s", error in=w773, w769) -> (resulting string=w770:string, error out=w772:errorcluster)  [unwired: 1 in]
        }
        frame "Is In Packed Library" {
          n201 = property class="VI"(reference=w783, error in=w784) -> (error out=w781:errorcluster, "IsInPackedLibrary"=w777:bool)  [unwired: 1 out]
          n202 = Format Into String(format string="%s", error in=w781, w777) -> (resulting string=w778:string, error out=w780:errorcluster)  [unwired: 1 in]
        }
        frame "Is Instance" {
          n203 = property class="VI"(reference=w791, error in=w792) -> (error out=w789:errorcluster, "Is Instance ?"=w785:bool)  [unwired: 1 out]
          n204 = Format Into String(format string="%s", error in=w789, w785) -> (resulting string=w786:string, error out=w788:errorcluster)  [unwired: 1 in]
        }
        frame "Is Probe" {
          n205 = property class="VI"(reference=w799, error in=w800) -> (error out=w797:errorcluster, "IsSmartProbe"=w793:bool)  [unwired: 1 out]
          n206 = Format Into String(format string="%s", error in=w797, w793) -> (resulting string=w794:string, error out=w796:errorcluster)  [unwired: 1 in]
        }
        frame "Is Running Interactively" {
          n207 = property class="VI"(reference=w807, error in=w808) -> (error out=w805:errorcluster, "HasRemoteObservers"=w801:bool)  [unwired: 1 out]
          n208 = Format Into String(format string="%s", error in=w805, w801) -> (resulting string=w802:string, error out=w804:errorcluster)  [unwired: 1 in]
        }
        frame "Is Skinned" {
          n209 = property class="VI"(reference=w815, error in=w816) -> (error out=w813:errorcluster, "IsSkinned"=w809:bool)  [unwired: 1 out]
          n210 = Format Into String(format string="%s", error in=w813, w809) -> (resulting string=w810:string, error out=w812:errorcluster)  [unwired: 1 in]
        }
        frame "Is System VI" {
          n211 = property class="VI"(reference=w823, error in=w824) -> (error out=w821:errorcluster, "IsSystemVI"=w817:bool)  [unwired: 1 out]
          n212 = Format Into String(format string="%s", error in=w821, w817) -> (resulting string=w818:string, error out=w820:errorcluster)  [unwired: 1 in]
        }
        frame "Is VI Paused?" {
          n213 = property class="VI"(reference=w831, error in=w832) -> (error out=w829:errorcluster, "Is VI Paused?"=w825:bool)  [unwired: 1 out]
          n214 = Format Into String(format string="%s", error in=w829, w825) -> (resulting string=w826:string, error out=w828:errorcluster)  [unwired: 1 in]
        }
        frame "Is XNode VI" {
          n215 = property class="VI"(reference=w839, error in=w840) -> (error out=w837:errorcluster, "X VI"=w833:bool)  [unwired: 1 out]
          n216 = Format Into String(format string="%s", error in=w837, w833) -> (resulting string=w834:string, error out=w836:errorcluster)  [unwired: 1 in]
        }
        frame "Item ID" {
          n217 = property class="VI"(reference=w847, error in=w848) -> (error out=w845:errorcluster, "ItemID"=w841:string)  [unwired: 1 out]
          n218 = Format Into String(format string="%s", error in=w845, w841) -> (resulting string=w842:string, error out=w844:errorcluster)  [unwired: 1 in]
        }
        frame "Ladder VI Needs Scripting" {
          n219 = property class="VI"(reference=w855, error in=w856) -> (error out=w853:errorcluster, "LadderVINeedsScripting"=w849:bool)  [unwired: 1 out]
          n220 = Format Into String(format string="%s", error in=w853, w849) -> (resulting string=w850:string, error out=w852:errorcluster)  [unwired: 1 in]
        }
        frame "Library:Version" {
          n221 = property class="VI"(reference=w867, error in=w868) -> (error out=w865:errorcluster, "Library.Version"=w861:T12)  [unwired: 1 out]
          n222 = Unbundle By Name(w861) -> ("Major"=w860:u16, "Minor"=w859:u16, "Fix"=w858:u16, "Build"=w857:u16)
          n223 = Format Into String(format string="%d.%d.%d.%d", error in=w865, w860, w859, w858, w857) -> (resulting string=w862:string, error out=w864:errorcluster)  [unwired: 1 in]
        }
        frame "Metrics:Block Diagram Loaded" {
          n224 = property class="VI"(reference=w875, error in=w876) -> (error out=w873:errorcluster, "DiagramLoaded"=w869:bool)  [unwired: 1 out]
          n225 = Format Into String(format string="%s", error in=w873, w869) -> (resulting string=w870:string, error out=w872:errorcluster)  [unwired: 1 in]
        }
        frame "Metrics:Code Size" {
          n226 = property class="VI"(reference=w883, error in=w884) -> (error out=w881:errorcluster, "Metric.CodeSize"=w877:u32)  [unwired: 1 out]
          n227 = Format Into String(format string="%d", error in=w881, w877) -> (resulting string=w878:string, error out=w880:errorcluster)  [unwired: 1 in]
        }
        frame "Metrics:Front Panel Loaded" {
          n228 = property class="VI"(reference=w891, error in=w892) -> (error out=w889:errorcluster, "PanelLoaded"=w885:bool)  [unwired: 1 out]
          n229 = Format Into String(format string="%s", error in=w889, w885) -> (resulting string=w886:string, error out=w888:errorcluster)  [unwired: 1 in]
        }
        frame "Metrics:Number of clones" {
          n230 = property class="VI"(reference=w899, error in=w900) -> (error out=w897:errorcluster, "Metric.NumberOfClones"=w893:u32)  [unwired: 1 out]
          n231 = Format Into String(format string="%d", error in=w897, w893) -> (resulting string=w894:string, error out=w896:errorcluster)  [unwired: 1 in]
        }
        frame "Metrics:Size of Block Diagram" {
          n232 = property class="VI"(reference=w907, error in=w908) -> (error out=w905:errorcluster, "Metric.BDSize"=w901:u32)  [unwired: 1 out]
          n233 = Format Into String(format string="%d", error in=w905, w901) -> (resulting string=w902:string, error out=w904:errorcluster)  [unwired: 1 in]
        }
        frame "Metrics:Size of Front Panel" {
          n234 = property class="VI"(reference=w915, error in=w916) -> (error out=w913:errorcluster, "Metric.FPSize"=w909:u32)  [unwired: 1 out]
          n235 = Format Into String(format string="%d", error in=w913, w909) -> (resulting string=w910:string, error out=w912:errorcluster)  [unwired: 1 in]
        }
        frame "Metrics:Total Data Size" {
          n236 = property class="VI"(reference=w923, error in=w924) -> (error out=w921:errorcluster, "Metric.DataSize"=w917:u32)  [unwired: 1 out]
          n237 = Format Into String(format string="%d", error in=w921, w917) -> (resulting string=w918:string, error out=w920:errorcluster)  [unwired: 1 in]
        }
        frame "Modifications:Block Diagram Mods Bitset" {
          n238 = property class="VI"(reference=w931, error in=w932) -> (error out=w929:errorcluster, "Mods.Block Diagram"=w925:u32)  [unwired: 1 out]
          n239 = Format Into String(format string="%d", error in=w929, w925) -> (resulting string=w926:string, error out=w928:errorcluster)  [unwired: 1 in]
        }
        frame "Modifications:Front Panel Mods Bitset" {
          n240 = property class="VI"(reference=w939, error in=w940) -> (error out=w937:errorcluster, "Mods.Front Panel"=w933:u32)  [unwired: 1 out]
          n241 = Format Into String(format string="%d", error in=w937, w933) -> (resulting string=w934:string, error out=w936:errorcluster)  [unwired: 1 in]
        }
        frame "Modifications:User Changes" {
          n242 = property class="VI"(reference=w947, error in=w948) -> (error out=w945:errorcluster, "Mods.User Changes"=w941:bool)  [unwired: 1 out]
          n243 = Format Into String(format string="%s", error in=w945, w941) -> (resulting string=w942:string, error out=w944:errorcluster)  [unwired: 1 in]
        }
        frame "Modifications:VI Modifications Bitset" {
          n244 = property class="VI"(reference=w955, error in=w956) -> (error out=w953:errorcluster, "Mods.VI"=w949:u64)  [unwired: 1 out]
          n245 = Format Into String(format string="%d", error in=w953, w949) -> (resulting string=w950:string, error out=w952:errorcluster)  [unwired: 1 in]
        }
        frame "No Clone If Instance VI" {
          n246 = property class="VI"(reference=w963, error in=w964) -> (error out=w961:errorcluster, "NoCloneIfInstanceVI"=w957:bool)  [unwired: 1 out]
          n247 = Format Into String(format string="%s", error in=w961, w957) -> (resulting string=w958:string, error out=w960:errorcluster)  [unwired: 1 in]
        }
        frame "Number of Non-Proxy Callers" {
          n248 = property class="VI"(reference=w971, error in=w972) -> (error out=w969:errorcluster, "NonProxyCallers"=w965:i32)  [unwired: 1 out]
          n249 = Format Into String(format string="%d", error in=w969, w965) -> (resulting string=w966:string, error out=w968:errorcluster)  [unwired: 1 in]
        }
        frame "Printing:Block Diagram Scaling?" {
          n250 = property class="VI"(reference=w979, error in=w980) -> (error out=w977:errorcluster, "Printing.BDScaling"=w973:bool)  [unwired: 1 out]
          n251 = Format Into String(format string="%s", error in=w977, w973) -> (resulting string=w974:string, error out=w976:errorcluster)  [unwired: 1 in]
        }
        frame "Printing:Front Panel Scaling?" {
          n252 = property class="VI"(reference=w987, error in=w988) -> (error out=w985:errorcluster, "Printing.FPScaling"=w981:bool)  [unwired: 1 out]
          n253 = Format Into String(format string="%s", error in=w985, w981) -> (resulting string=w982:string, error out=w984:errorcluster)  [unwired: 1 in]
        }
        frame "Printing:Header Content:Date Printed?" {
          n254 = property class="VI"(reference=w995, error in=w996) -> (error out=w993:errorcluster, "Print.Header Content.Date Printed"=w989:bool)  [unwired: 1 out]
          n255 = Format Into String(format string="%s", error in=w993, w989) -> (resulting string=w990:string, error out=w992:errorcluster)  [unwired: 1 in]
        }
        frame "Printing:Header Content:Modify Date?" {
          n256 = property class="VI"(reference=w1003, error in=w1004) -> (error out=w1001:errorcluster, "Print.Header Content.Modify Date"=w997:bool)  [unwired: 1 out]
          n257 = Format Into String(format string="%s", error in=w1001, w997) -> (resulting string=w998:string, error out=w1000:errorcluster)  [unwired: 1 in]
        }
        frame "Printing:Header Content:Page Number?" {
          n258 = property class="VI"(reference=w1011, error in=w1012) -> (error out=w1009:errorcluster, "Print.Header Content.Page Number"=w1005:bool)  [unwired: 1 out]
          n259 = Format Into String(format string="%s", error in=w1009, w1005) -> (resulting string=w1006:string, error out=w1008:errorcluster)  [unwired: 1 in]
        }
        frame "Printing:Header Content:VI Icon?" {
          n260 = property class="VI"(reference=w1019, error in=w1020) -> (error out=w1017:errorcluster, "Print.Header Content.VIIcon"=w1013:bool)  [unwired: 1 out]
          n261 = Format Into String(format string="%s", error in=w1017, w1013) -> (resulting string=w1014:string, error out=w1016:errorcluster)  [unwired: 1 in]
        }
        frame "Printing:Header Content:VI Name?" {
          n262 = property class="VI"(reference=w1027, error in=w1028) -> (error out=w1025:errorcluster, "Printing.HeaderContent.VIName"=w1021:bool)  [unwired: 1 out]
          n263 = Format Into String(format string="%s", error in=w1025, w1021) -> (resulting string=w1022:string, error out=w1024:errorcluster)  [unwired: 1 in]
        }
        frame "Printing:Header Content:VI Path?" {
          n264 = property class="VI"(reference=w1035, error in=w1036) -> (error out=w1033:errorcluster, "Printing.Header Content.VIPath"=w1029:bool)  [unwired: 1 out]
          n265 = Format Into String(format string="%s", error in=w1033, w1029) -> (resulting string=w1030:string, error out=w1032:errorcluster)  [unwired: 1 in]
        }
        frame "Printing:Margins" {
          n266 = property class="VI"(reference=w1048, error in=w1049) -> (error out=w1046:errorcluster, "Printing.Margin"=w1042:T13)  [unwired: 1 out]
          n267 = Unbundle By Name(w1042) -> ("Top"=w1040:sgl, "Left"=w1041:sgl, "Bottom"=w1038:sgl, "Right"=w1039:sgl, "Measurement System"=w1037:enum8{"Inches", "cm"})
          n268 = Format Into String(format string="{L:%#g, T:%#g, R:%#g, B:%#g, U:%s}", error in=w1046, w1041, w1040, w1039, w1038, w1037) -> (resulting string=w1043:string, error out=w1045:errorcluster)  [unwired: 1 in]
        }
        frame "Printing:Page Headers?" {
          n269 = property class="VI"(reference=w1056, error in=w1057) -> (error out=w1054:errorcluster, "Printing.Headers"=w1050:bool)  [unwired: 1 out]
          n270 = Format Into String(format string="%s", error in=w1054, w1050) -> (resulting string=w1051:string, error out=w1053:errorcluster)  [unwired: 1 in]
        }
        frame "Printing:Page Orientation" {
          n271 = property class="VI"(reference=w1064, error in=w1065) -> (error out=w1062:errorcluster, "Printing.Orientation"=w1058:T14)  [unwired: 1 out]
          n272 = Format Into String(format string="%s", error in=w1062, w1058) -> (resulting string=w1059:string, error out=w1061:errorcluster)  [unwired: 1 in]
        }
        frame "Purgative" {
          n273 = property class="VI"(reference=w1072, error in=w1073) -> (error out=w1070:errorcluster, "Purgative"=w1066:bool)  [unwired: 1 out]
          n274 = Format Into String(format string="%s", error in=w1070, w1066) -> (resulting string=w1067:string, error out=w1069:errorcluster)  [unwired: 1 in]
        }
        frame "Run-Time Menu Path" {
          n275 = property class="VI"(reference=w1080, error in=w1081) -> (error out=w1078:errorcluster, "RT Menu Path"=w1074:path)  [unwired: 1 out]
          n276 = Format Into String(format string="%s", error in=w1078, w1074) -> (resulting string=w1075:string, error out=w1077:errorcluster)  [unwired: 1 in]
        }
        frame "Saved Version" {
          n277 = property class="VI"(reference=w1088, error in=w1089) -> (error out=w1086:errorcluster, "SavedVersion"=w1082:u32)  [unwired: 1 out]
          n278 = Format Into String(format string="%d", error in=w1086, w1082) -> (resulting string=w1083:string, error out=w1085:errorcluster)  [unwired: 1 in]
        }
        frame "Statechart:Is Sub Panel Editable" {
          n279 = property class="VI"(reference=w1096, error in=w1097) -> (error out=w1094:errorcluster, "IsSCEditable"=w1090:bool)  [unwired: 1 out]
          n280 = Format Into String(format string="%s", error in=w1094, w1090) -> (resulting string=w1091:string, error out=w1093:errorcluster)  [unwired: 1 in]
        }
        frame "Statechart:Supress Parse" {
          n281 = property class="VI"(reference=w1104, error in=w1105) -> (error out=w1102:errorcluster, "SuppressSCParse"=w1098:bool)  [unwired: 1 out]
          n282 = Format Into String(format string="%s", error in=w1102, w1098) -> (resulting string=w1099:string, error out=w1101:errorcluster)  [unwired: 1 in]
        }
        frame "Suppress Data Manager" {
          n283 = property class="VI"(reference=w1112, error in=w1113) -> (error out=w1110:errorcluster, "SuppressDataMgr"=w1106:bool)  [unwired: 1 out]
          n284 = Format Into String(format string="%s", error in=w1110, w1106) -> (resulting string=w1107:string, error out=w1109:errorcluster)  [unwired: 1 in]
        }
        frame "Suppress Instance VI Halo" {
          n285 = property class="VI"(reference=w1120, error in=w1121) -> (error out=w1118:errorcluster, "SuppInstVIHalo"=w1114:bool)  [unwired: 1 out]
          n286 = Format Into String(format string="%s", error in=w1118, w1114) -> (resulting string=w1115:string, error out=w1117:errorcluster)  [unwired: 1 in]
        }
        frame "Suppress Transact Info" {
          n287 = property class="VI"(reference=w1128, error in=w1129) -> (error out=w1126:errorcluster, "SuppressTransactInfo"=w1122:bool)  [unwired: 1 out]
          n288 = Format Into String(format string="%s", error in=w1126, w1122) -> (resulting string=w1123:string, error out=w1125:errorcluster)  [unwired: 1 in]
        }
        frame "Suppress Type Prop" {
          n289 = property class="VI"(reference=w1136, error in=w1137) -> (error out=w1134:errorcluster, "NoTypeProp"=w1130:bool)  [unwired: 1 out]
          n290 = Format Into String(format string="%s", error in=w1134, w1130) -> (resulting string=w1131:string, error out=w1133:errorcluster)  [unwired: 1 in]
        }
        frame "Tagged And Not Edited" {
          n291 = property class="VI"(reference=w1144, error in=w1145) -> (error out=w1142:errorcluster, "TaggedAndNotEdited"=w1138:bool)  [unwired: 1 out]
          n292 = Format Into String(format string="%s", error in=w1142, w1138) -> (resulting string=w1139:string, error out=w1141:errorcluster)  [unwired: 1 in]
        }
        frame "Terminal Bounds[]" {
          n293 = property class="VI"(reference=w1161, error in=w1162) -> (error out=w1159:errorcluster, "TermBnds[]"=w1157:T4[])  [unwired: 1 out]
          n294 = for {
            tunnel: w1157 -> [w1168] mode=indexing
            shift-right: [w1170] -> w1158
            shift-left: w1159 -> [w1171]
            tunnel: [w1163] -> w1146 mode=indexing
            n295 = Unbundle By Name(w1168) -> ("Left"=w1167:i16, "Top"=w1166:i16, "Right"=w1165:i16, "Bottom"=w1164:i16)
            n296 = Format Into String(format string="{L:%d, T:%d, R:%d, B:%d}", error in=w1171, w1167, w1166, w1165, w1164) -> (resulting string=w1163:string, error out=w1170:errorcluster)  [unwired: 1 in]
          }
          n297 = Delete From Array(array=w1146) -> (deleted portion=w1151:string, array with subset deleted=w1154:string[])  [unwired: 2 in]
          n298 = Array Size(array=w1154) -> (size(s)=w1156:i32)
          n299 = Initialize Array(", ", w1156) -> (w1153:string[])
          n300 = Interleave 1D Arrays(w1154, w1153) -> (w1152:string[])
          n301 = Concatenate Strings(w1152, w1151) -> (w1149:string)
          n302 = Format Into String(format string="[%s]", error in=w1158, w1149) -> (resulting string=w1148:string, error out=w1150:errorcluster)  [unwired: 1 in]
        }
        frame "Tool Bar:Show Abort Button" {
          n303 = property class="VI"(reference=w1178, error in=w1179) -> (error out=w1176:errorcluster, "TB.ShowAbortBut"=w1172:bool)  [unwired: 1 out]
          n304 = Format Into String(format string="%s", error in=w1176, w1172) -> (resulting string=w1173:string, error out=w1175:errorcluster)  [unwired: 1 in]
        }
        frame "Tool Bar:Show Free Run Button" {
          n305 = property class="VI"(reference=w1186, error in=w1187) -> (error out=w1184:errorcluster, "TB.ShowFreeRunBut"=w1180:bool)  [unwired: 1 out]
          n306 = Format Into String(format string="%s", error in=w1184, w1180) -> (resulting string=w1181:string, error out=w1183:errorcluster)  [unwired: 1 in]
        }
        frame "Tool Bar:Show Run Button" {
          n307 = property class="VI"(reference=w1194, error in=w1195) -> (error out=w1192:errorcluster, "TB.ShowRunBut"=w1188:bool)  [unwired: 1 out]
          n308 = Format Into String(format string="%s", error in=w1192, w1188) -> (resulting string=w1189:string, error out=w1191:errorcluster)  [unwired: 1 in]
        }
        frame "Tool Bar:Visible" {
          n309 = property class="VI"(reference=w1202, error in=w1203) -> (error out=w1200:errorcluster, "TB.Visible"=w1196:bool)  [unwired: 1 out]
          n310 = Format Into String(format string="%s", error in=w1200, w1196) -> (resulting string=w1197:string, error out=w1199:errorcluster)  [unwired: 1 in]
        }
        frame "Tool Kit Attr" {
          n311 = property class="VI"(reference=w1213, error in=w1214) -> (error out=w1211:errorcluster, "ToolKitAttr"=w1207:T15)  [unwired: 1 out]
          n312 = Unbundle By Name(w1207) -> ("Creator"=w1206:string, "Toolkit"=w1205:string, "Version"=w1204:i32)
          n313 = Format Into String(format string="{C:%s, T:%s, V:%d}", error in=w1211, w1206, w1205, w1204) -> (resulting string=w1208:string, error out=w1210:errorcluster)  [unwired: 1 in]
        }
        frame "VI Clone Name" {
          n314 = property class="VI"(reference=w1221, error in=w1222) -> (error out=w1219:errorcluster, "Clone Name"=w1215:string)  [unwired: 1 out]
          n315 = Format Into String(format string="%s", error in=w1219, w1215) -> (resulting string=w1216:string, error out=w1218:errorcluster)  [unwired: 1 in]
        }
        frame "VI Compile Time" {
          n316 = property class="VI"(reference=w1229, error in=w1230) -> (error out=w1227:errorcluster, "Compile Time"=w1223:i32)  [unwired: 1 out]
          n317 = Format Into String(format string="%d", error in=w1227, w1223) -> (resulting string=w1224:string, error out=w1226:errorcluster)  [unwired: 1 in]
        }
        frame "VI Description" {
          n318 = property class="VI"(reference=w1237, error in=w1238) -> (error out=w1235:errorcluster, "Description"=w1231:string)  [unwired: 1 out]
          n319 = Format Into String(format string="%s", error in=w1235, w1231) -> (resulting string=w1232:string, error out=w1234:errorcluster)  [unwired: 1 in]
        }
        frame "VI Linker Errors" {
          n320 = property class="VI"(reference=w1245, error in=w1246) -> (error out=w1243:errorcluster, "VILoadErr"=w1239:string)  [unwired: 1 out]
          n321 = Format Into String(format string="%s", error in=w1243, w1239) -> (resulting string=w1240:string, error out=w1242:errorcluster)  [unwired: 1 in]
        }
        frame "VI Name" {
          n322 = property class="VI"(reference=w1253, error in=w1254) -> (error out=w1251:errorcluster, "Name"=w1247:string)  [unwired: 1 out]
          n323 = Format Into String(format string="%s", error in=w1251, w1247) -> (resulting string=w1248:string, error out=w1250:errorcluster)  [unwired: 1 in]
        }
        frame "VI Path" {
          n324 = property class="VI"(reference=w1261, error in=w1262) -> (error out=w1259:errorcluster, "Path"=w1255:path)  [unwired: 1 out]
          n325 = Format Into String(format string="%s", error in=w1259, w1255) -> (resulting string=w1256:string, error out=w1258:errorcluster)  [unwired: 1 in]
        }
        frame "VI Type" {
          n326 = property class="VI"(reference=w1269, error in=w1270) -> (error out=w1267:errorcluster, "VIType"=w1263:T16)  [unwired: 1 out]
          n327 = Format Into String(format string="%s", error in=w1267, w1263) -> (resulting string=w1264:string, error out=w1266:errorcluster)  [unwired: 1 in]
        }
      }
      n328 = Compound Arithmetic op=AND(w8, invert w9) -> (w7:bool)
      n329 = Select(t=w12, s=w9, f=w9) -> (s? t:f=w11:errorcluster)
    }
    frame Error {
    }
  }
  "error out" <- w2
  "Value" <- w1
  "Supported?" <- w3
  "VI Refnum out" <- "VI Refnum in"
